vi "StructuredDataToVariant.vi"(7 "Data Type":variant, 8 "error in (no error)":errorcluster, 10 "StructuredData":variant, 11 "BlueJSONTextSerializer in":refnum<class "BlueJSONTextSerializer.lvclass">) -> (0 "error out":errorcluster, 2 "Variant":variant, 3 "BlueJSONTextSerializer out":refnum<class "BlueJSONTextSerializer.lvclass">)   [LabVIEW 2019, in "BlueJSONTextSerializer.lvlib" / "BlueJSONTextSerializer.lvclass"]
uses:
  BlueJSONTextSerializer.lvclass
  StructuredData.ctl
  <vilib>/JDP Science/JSONtext/JSONtext.lvlib
  BlueJSONtext LVClass Serializer/BlueJSONtext LVClass Serializer.lvclass
  C:/Program Files (x86)/National Instruments/LabVIEW 2019/vi.lib/JDP Science/JSONtext/LVClass Serializer/JSONtext LVClass Serializer.lvclass
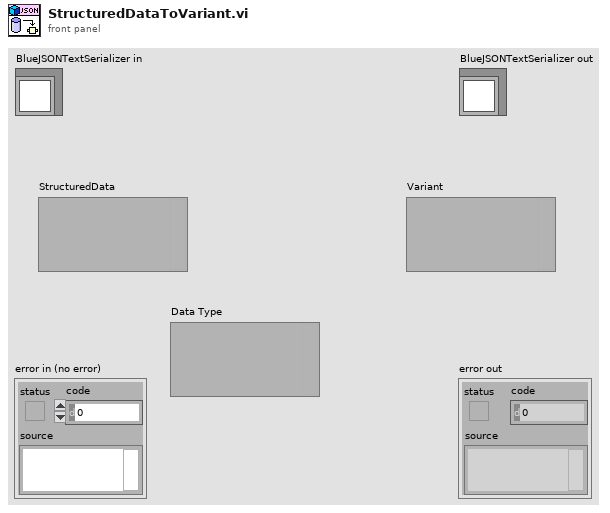
[diagram p1: front panel]
types:
  T1 = typedef "BlueJSONTextSerializer.lvlib/BlueJSONTextSerializer.lvclass/StructuredData.ctl" = cluster{"JSON":string, "Offset":i32}
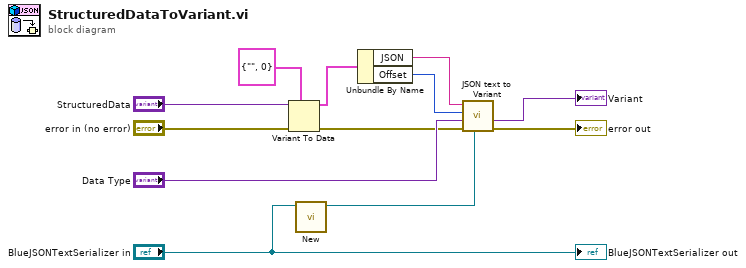
[diagram p0: block diagram]
diagram:
  n1 = Variant To Data(error in="error in (no error)", type=T1 {"JSON"="", "Offset"=0} ("Cluster"), Variant="StructuredData") -> (data=w9:T1, error out=w5:errorcluster)
  n2 = call "New.vi"("BlueJSONTextSerializer"="BlueJSONTextSerializer in") -> ("BlueJSONtext LVClass Serializer out"=w1:refnum<class "BlueJSONtext LVClass Serializer.lvclass">)  [unwired: 10 in]
  n3 = Unbundle By Name(w9) -> ("JSON"=w8:string, "Offset"=w7:i32)
  n4 = call <vilib>:"JSON text to Variant.vi"("LVClass Serializer"=w1, "error in (no error)"=w5, "Data Type"="Data Type", "Offset"=w7, "JSON"=w8) -> ("error out"=→"error out":errorcluster, "Variant out"=→"Variant":variant)  [unwired: 5 in]
  "BlueJSONTextSerializer out" <- "BlueJSONTextSerializer in"
